vi "Save As EDF.vi"(10 "iMode":i32, 11 "szPath":string) -> (2 "function return":u32, 3 "szPath out":string)   [LabVIEW 2018, in "AndorSDK.lvlib"]
doc: "EXPNETTYPE unsigned int WINAPI SaveAsEDF(char * szPath, int iMode);"
uses:
  AndorSDK.lvlib
  ATMCD32D.dll
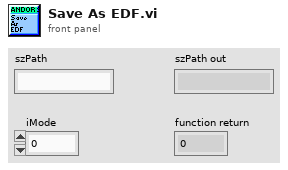
[diagram p1: front panel]
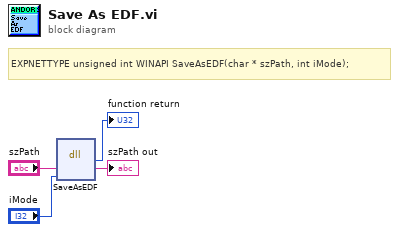
[diagram p0: block diagram]
diagram:
  # "EXPNETTYPE unsigned int WINAPI SaveAsEDF(char * szPath, int iMode);"
  n1 = dll-call lib="PTH2babs E\nPersönliches02 - Arbeit03-HiwijobsLabviewCodelibANDOR\tAndor SDK\nATMCD32D.*" fn="SaveAsEDF"("szPath"="szPath", "iMode"="iMode") -> (→"function return":u32, "szPath"=→"szPath out":string)  [unwired: 4 in, 2 out]
